vi "AddFailure.vi"(7 "Time":dbl, 8 "error in (no error)":errorcluster, 9 "Failure":errorcluster, 10 "Test":refnum<class "Test.lvclass">, 11 "TestResult in":refnum<class "TestResult.lvclass">) -> (0 "error out":errorcluster, 3 "TestResult out":refnum<class "TestResult.lvclass">)   [LabVIEW 2019, in "TestResult.lvclass"]
doc: "Adds a failure to the list of failures."
uses:
  TestResult.lvclass
  Test/Test.lvclass
  TestResult.lvclass/TestResult.ctl
  TestListener/TestListener.lvclass
  TestFailure/TestFailure.lvclass
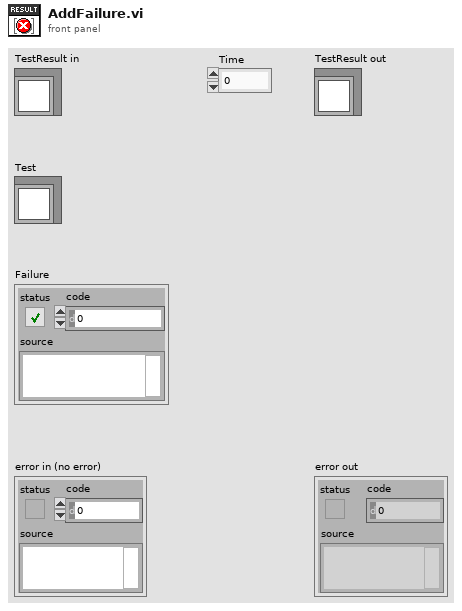
[diagram p1: front panel]
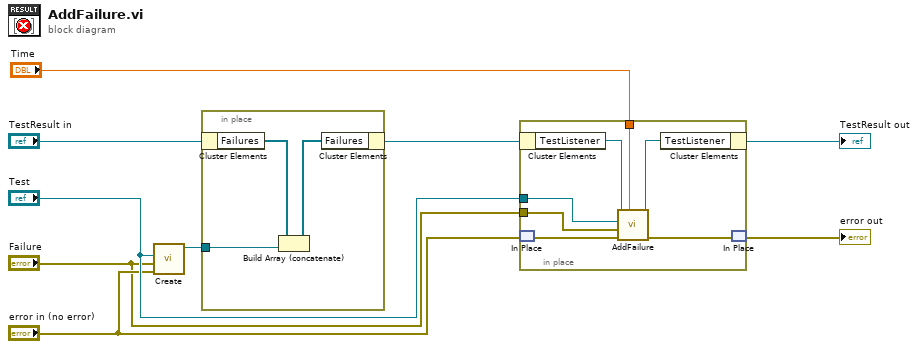
[diagram p0: block diagram]
diagram:
  n1 = call "Create.vi"("error in (no error)"="error in (no error)", "Failure"="Failure", "Test"="Test") -> ("TestFailure"=w9:refnum<class "TestFailure.lvclass">)  [unwired: 7 in, 1 out]
  n2 = in-place {
    in-place-border: w9 -> [w10]
    n3 = in-place-cluster #1("TestResult in") -> ("Failures"=w12:refnum<class "TestFailure.lvclass">[])
    n4 = Build Array (concatenate)(w12, w10) -> (w11:refnum<class "TestFailure.lvclass">[])
    n5 = in-place-cluster #1("Failures"=w11) -> (w7:refnum<class "TestResult.lvclass">)
  }
  n6 = in-place {
    in-place-border: "Test" -> [w19]
    in-place-border: "Time" -> [w14]
    in-place-border: "Failure" -> [w13]
    n7 = in-place-cluster #2(w7) -> ("TestListener"=w16:refnum<class "TestListener.lvclass">)
    n8 = in-place-match #3("error in (no error)") -> (w18:errorcluster)
    n9 = call-dynamic "AddFailure.vi"("Time"=w14, "error in (no error)"=w18, "Failure"=w13, "Test"=w19, "TestListener in"=w16) -> ("error out"=w17:errorcluster, "TestListener out"=w15:refnum<class "TestListener.lvclass">)  [unwired: 5 in]
    n10 = in-place-cluster #2("TestListener"=w15) -> (→"TestResult out":refnum<class "TestResult.lvclass">)
    n11 = in-place-match #3(w17) -> (→"error out":errorcluster)
  }
